vi "FFT.vi"() -> ()   [LabVIEW 2020]
uses:
  <vilib>/rvi/Analysis/measure/FFT/simModelSupport/niFPGA FFT Outside SCTL Sim Properties.ctl
  <vilib>/rvi/Analysis/measure/FFT/simModelSupport/niFPGA FFT Sim Types.ctl
  <vilib>/rvi/Analysis/measure/FFT/simModelSupport/niFpgaFFTSimArithmeticProperties.ctl
  <vilib>/rvi/Analysis/measure/FFT/simModelSupport/niFpgaFFTSimDfxp.ctl
  <vilib>/fxp/LVFixedPointQuantizationPolicyTypeDef.ctl
  <vilib>/rvi/FXPMathLib/FxpAtan2/subVIs/nifxpmath_Atan2_SimConfig.ctl
  <vilib>/rvi/FXPMathLib/FxpSinAndCos/subVIs/nifxpmath_SinAndCos_SimConfig.ctl
  <vilib>/rvi/DataTransferAndStorage/Container/Common/niFpgaContainerGetUniqueNameForEmu.vi
  <vilib>/rvi/DataTransferAndStorage/Container/Common/niFpgaContainerSetEmuInfo.vi
  <vilib>/rvi/eio/common/nirviEmuReportErrorAndStop.vi
  <vilib>/rvi/interface/RandomDataEmulation/niFpgaRandomDataHandleErrors.vi
  <vilib>/rvi/DataTransferAndStorage/Container/Common/niFpgaContainerExecOnDevCompGetState.vi
  <vilib>/rvi/Emulation/niFpgaEmulationIsFPGAContextNoSignature.vi
  <vilib>/rvi/Emulation/niFpgaSctlEmulationGetInTimedLoop.vi
  <vilib>/rvi/errors/niFpgaSetErrorForExecOnDevCompSimple.vi
  <vilib>/rvi/FIFO/Fifo_Resource/nirvififoEmulationSetSize.vi
  <vilib>/rvi/FIFO/Fifo_Resource/nirviFifoEmulationQueueMgr.vi
  <instcachedir>/0/nirviFifoEmulationQueueMgr_E5CAEC123FF24DC58D834DCA3CDAA9B5.lvgen/nirviFifoEmulationQueueMgr_E5CAEC123FF24DC58D834DCA3CDAA9B5_008.vi
  <vilib>/rvi/FIFO/Fifo_Resource/nirvififoEmulationDetermineInputValidOut.vi
  <vilib>/rvi/FIFO/Fifo_Resource/nirvififoEmulationCreateLock.vi
  <vilib>/rvi/Emulation/niFpgaProcessEmulError.vi
  <vilib>/rvi/FIFO/Fifo_Resource/nirvififoEmulationObtainLock.vi
  <vilib>/rvi/FIFO/Fifo_Resource/nirvififoEmulationReleaseLock.vi
  <vilib>/rvi/occurrence/nirviWaitOnOccurrenceBase.vi
  <vilib>/rvi/errors/nirviReportUnexpectedCaseInternalError.vi
  <vilib>/rvi/errors/nirviReportUnexpectedCaseInternalError (U32).vi
  <vilib>/Utility/error.llb/Clear Errors.vi
  <vilib>/rvi/Emulation/niFpgaGetClockAttributes.vi
  <vilib>/rvi/Emulation/niFpgaEmulationReportErrorSimple.vi
  <vilib>/rvi/Analysis/measure/FFT/simModelSupport/niFpgaFFTSimModelOutsideSCTLCore.vi
  <vilib>/rvi/FXPMathLib/FxpAtan2/simVIs/DllFxpAtan2Temp_sub.vi
  <instcachedir>/0/nirviFifoEmulationQueueMgr_E5CAEC123FF24DC58D834DCA3CDAA9B5.lvgen/nirviFifoEmulationQueueMgr_E5CAEC123FF24DC58D834DCA3CDAA9B5_002.vi
  <instcachedir>/0/nirviFifoEmulationQueueMgr_E5CAEC123FF24DC58D834DCA3CDAA9B5.lvgen/nirviFifoEmulationQueueMgr_E5CAEC123FF24DC58D834DCA3CDAA9B5_004.vi
  <vilib>/rvi/Emulation/niFpgaCriticalErrorInLSC.vi
  <vilib>/rvi/FXPMathLib/FxpSinAndCos/simVIs/DllFxpSinAndCosTemp_sub.vi
  <instcachedir>/0/nirviFifoEmulationQueueMgr_E5CAEC123FF24DC58D834DCA3CDAA9B5.lvgen/nirviFifoEmulationQueueMgr_E5CAEC123FF24DC58D834DCA3CDAA9B5_015.vi
  <vilib>/rvi/LocalResourceManager/LocalResourceManager.xnode
  <vilib>/rvi/DataTransferAndStorage/Container/XNode/niFpgaContainer.xnode
  <vilib>/rvi/interface/RandomDataEmulation/nirviRandomDataFpgaReadWriteTemplate.vi
  <vilib>/rvi/FIFO/Fifo_Resource/niFpgaFifoEmulationRefIn.vi
  <vilib>/rvi/Analysis/measure/FFT/XNode/niFpgaFFT.xnode
  <vilib>/rvi/FXPMathLib/FxpAtan2/XNode/nifxpmath_Atan2.xnode
  <vilib>/rvi/FXPMathLib/FxpSinAndCos/XNode/nifxpmath_SinAndCos.xnode
panel:
  out "Numeric 3":i32
  out "Numeric":i32
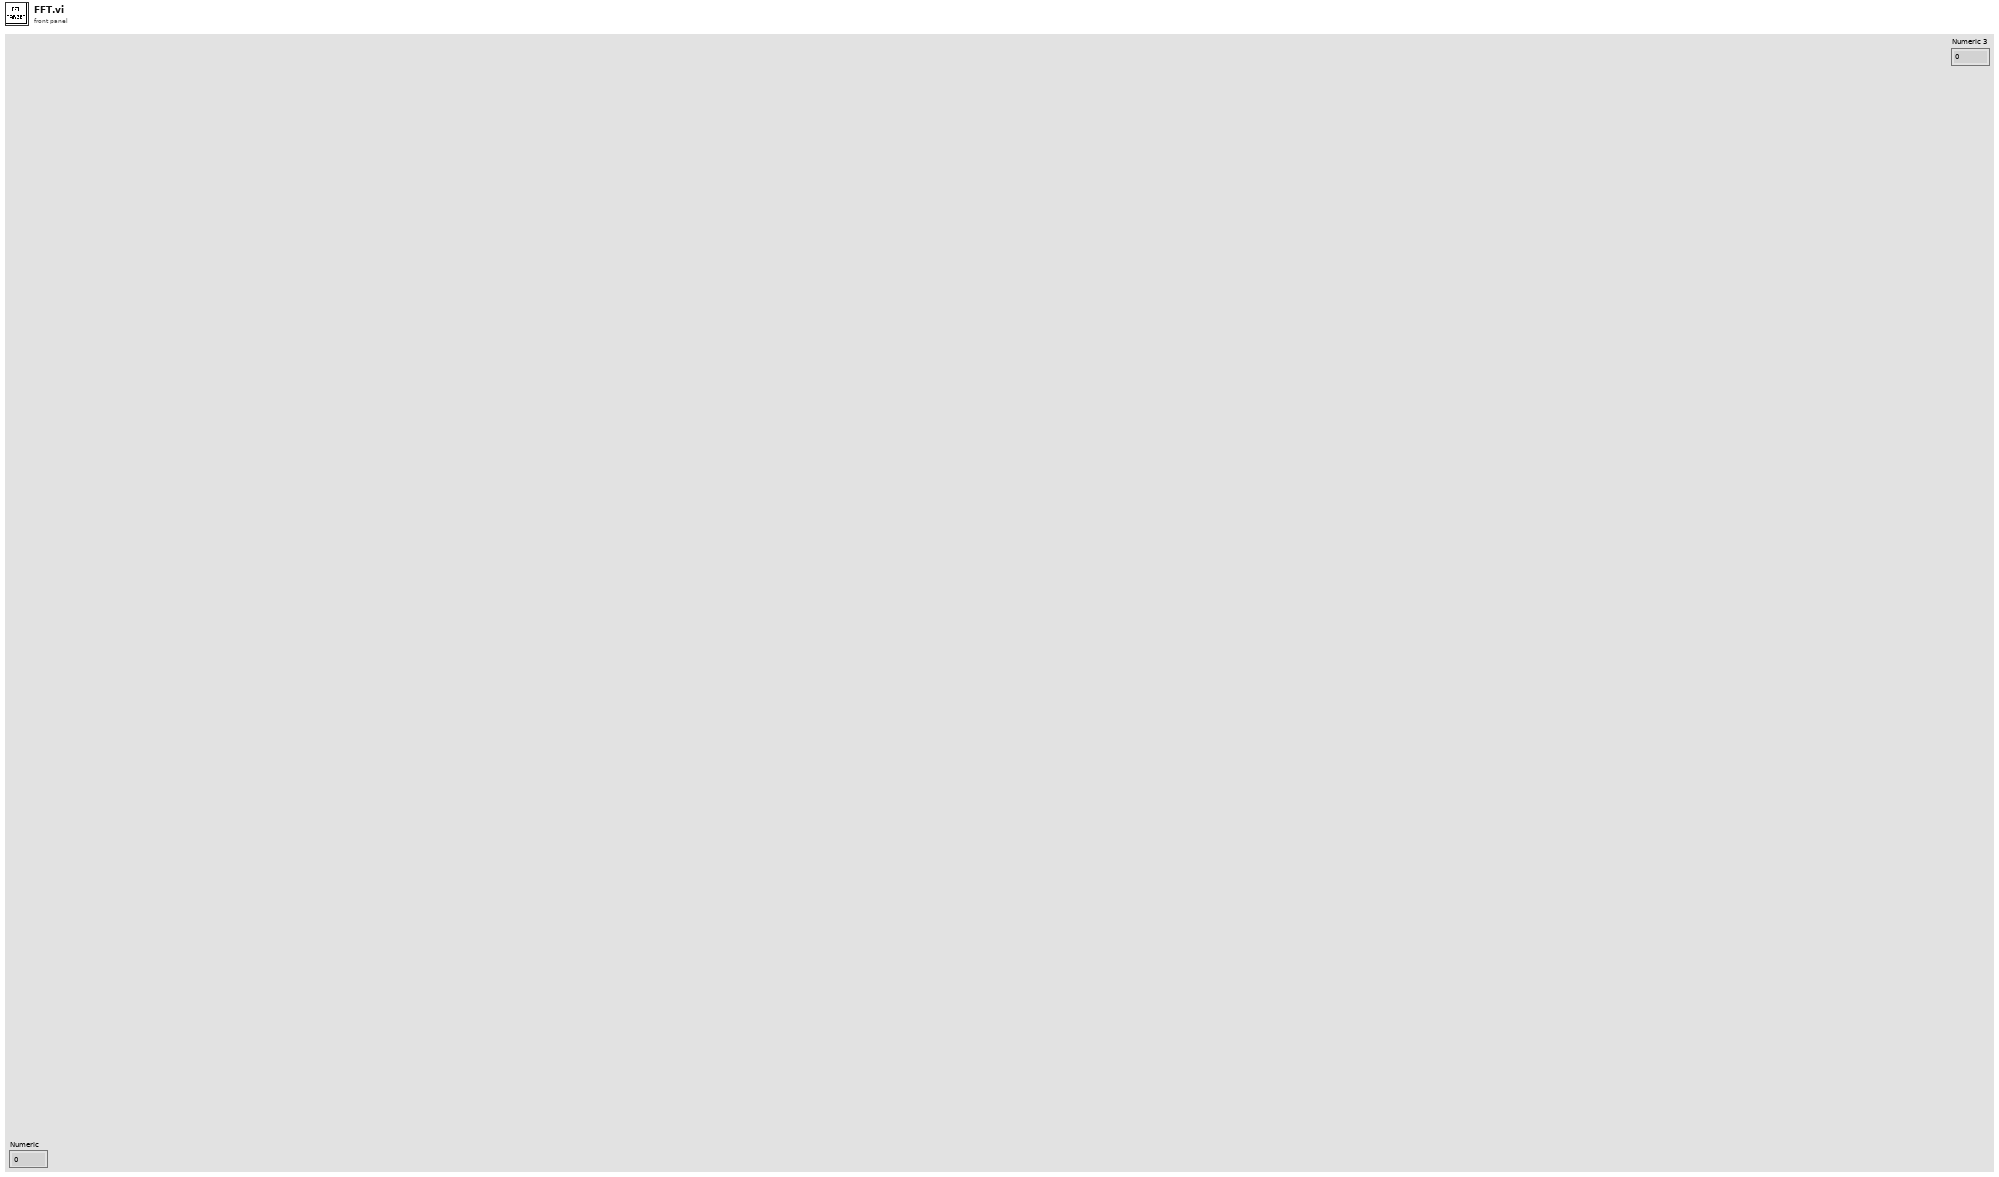
[diagram p1: front panel]
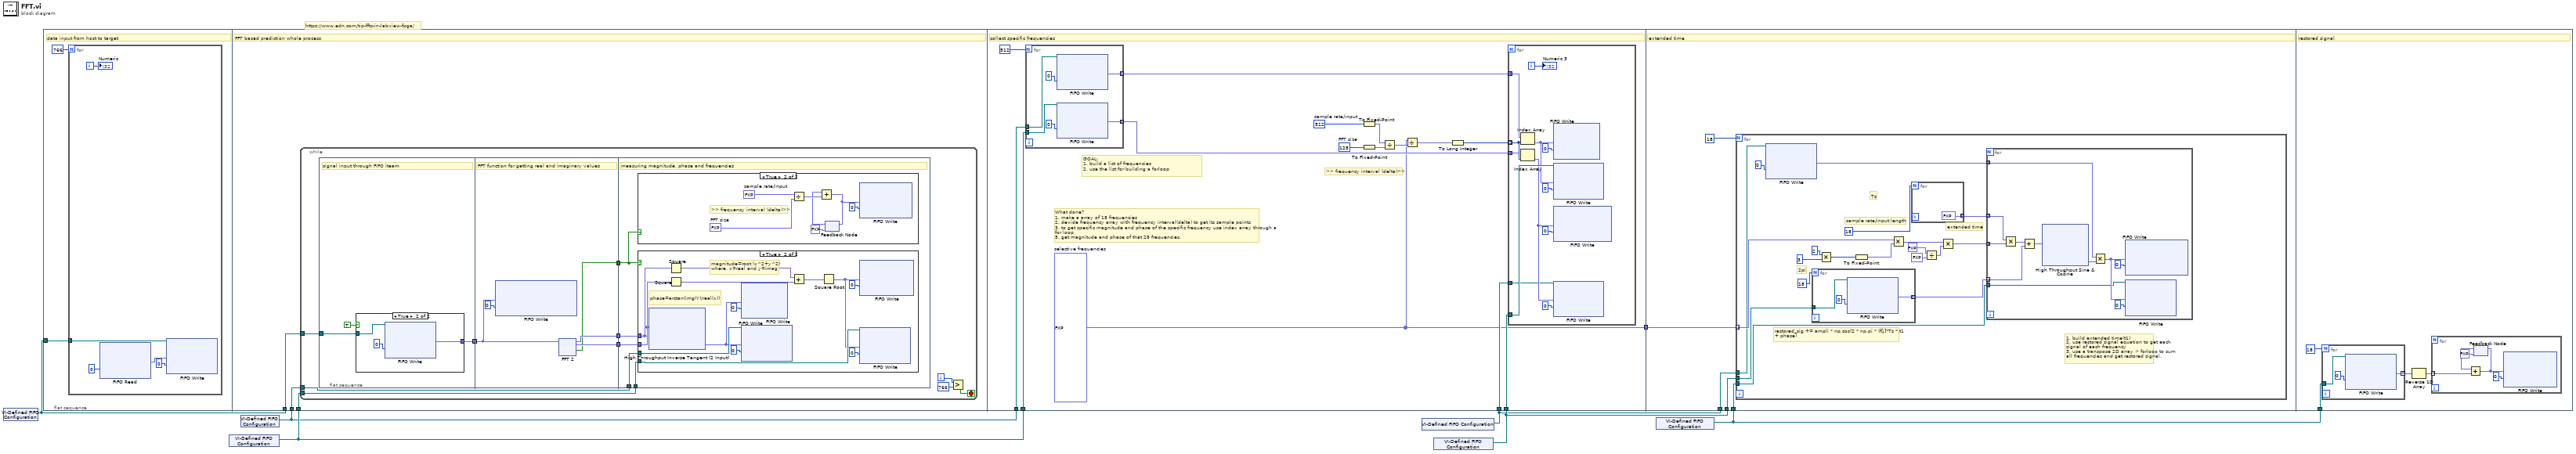
[diagram p0: block diagram]
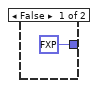
[diagram p2: hidden frame]
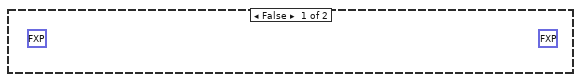
[diagram p4: hidden frame]
diagram:
  # "https://www.edn.com/tip-ffts-in-labview-fpga/"
  n1 = xnode "VI-Defined FIFO Configuration"() -> ("FIFO Out"=w7:refnum<k21>)
  n2 = flat-sequence {
    tunnel: w7 -> [w9]
    tunnel: w7 -> [w17]
    tunnel: w6 -> [w16]
    tunnel: w5 -> [w15]
    tunnel: w6 -> [w117]
    tunnel: w5 -> [w116]
    tunnel: w4 -> [w115]
    tunnel: w3 -> [w114]
    tunnel: [w113] -> w2
    tunnel: w4 -> [w150]
    tunnel: w3 -> [w149]
    tunnel: w2 -> [w148]
    tunnel: w1 -> [w147]
    tunnel: w1 -> [w218]
    frame #0 {
      # "data input from host to target"
      n3 = for {
        N: 766 -> [_]
        tunnel: w9 -> [w13]
        i -> [w10]
        n4 = xnode ("FIFO Read")("Timeout"=0) -> ("Element"=w11:fxp<+/-,24,7>)  [unwired: 1 in, 2 out]
        n5 = xnode ("FIFO Write")("Element"=w11, "Timeout"=0, "FIFO In"=w13) -> ()  [unwired: 2 out]
        "Numeric" <- w10
      }
    }
    frame #1 {
      # "FFT based prediction whole process"
      n6 = while {
        tunnel: w17 -> [w26]
        tunnel: w16 -> [w19]
        tunnel: w15 -> [w18]
        i -> [w25]
        stop <- w20 stop-if-true
        n7 = flat-sequence {
          tunnel: w26 -> [w30]
          tunnel: [w28] -> w24
          tunnel: w24 -> [w39]
          tunnel: [w38] -> w23
          tunnel: [w37] -> w22
          tunnel: [w36] -> w21
          tunnel: w23 -> [w63]
          tunnel: w22 -> [w62]
          tunnel: w21 -> [w64]
          tunnel: w19 -> [w61]
          tunnel: w18 -> [w60]
          frame #0 {
            # "signal input through FIFO iteam"
            n8 = case shown="True" TRUE {
              tunnel: w30 -> [_ w34]
              tunnel: [fxp<+/-,24,7> 0.0 ("Element") w32] -> w28
              frame False {
              }
              frame True {
                n9 = xnode ("FIFO Write")("Timeout"=0, "FIFO In"=w34) -> ("Element"=w32:fxp<+/-,24,7>)  [unwired: 2 out]
              }
            }
          }
          frame #1 {
            # "FFT function for getting real and imaginary values"
            n10 = xnode ("FIFO Write")("Element"=w39, "Timeout"=0) -> ()  [unwired: 1 in, 2 out]
            n11 = xnode ("FFT 2")("real data in"=w39) -> ("real data out"=w38:fxp<+/-,32,15>, "imaginary data out"=w37:fxp<+/-,32,15>, "output valid"=w36:bool)  [unwired: 2 in, 1 out]
          }
          frame #2 {
            # "measuring magnitude, phase and frequencies"
            n12 = case shown="True" w64 {
              frame False {
              }
              frame True {
                w66 = fxp<+,1,10> 512.0  # sample rate/input
                w65 = fxp<+,1,8> 128.0  # FFT size
                # ">> frequency interval (delta)>>"
                n13 = Divide(x=w66, y=w65) -> (x/y=w70:fxp<+/-,32,16>)
                n14 = feedback #1(fxp<+/-,32,16> 0.0) -> (w68:fxp<+/-,32,16>)
                n15 = Add(x=w68, y=w70) -> (x+y=w69:fxp<+/-,32,16>)
                n16 = feedback-in #1(w69) -> ()
                n17 = xnode ("FIFO Write")("Element"=w69, "Timeout"=0) -> ()  [unwired: 1 in, 2 out]
              }
            }
            n18 = case shown="True" w64 {
              tunnel: w62 -> [_ w74]
              tunnel: w63 -> [_ w73]
              tunnel: w61 -> [_ w78]
              tunnel: w60 -> [_ w75]
              frame False {
                (unwired) fxp<+/-,32,16> 0.0
                (unwired) fxp<+/-,32,16> 0.0
              }
              frame True {
                # "magnitude=root (x^2+y^2)\nwhere, x=real and y=imag"
                # "phase=arctan(img(Y)/real(x))"
                n19 = xnode "High Throughput Inverse Tangent (2 Input)"("y"=w74, "x"=w73) -> ("atan2(y,x) (pi)"=w72:fxp<+/-,16,2>)
                n20 = Square(x=w73) -> (x^2=w82:fxp<+,63,29>)
                n21 = Square(x=w74) -> (x^2=w77:fxp<+,63,29>)
                n22 = xnode ("FIFO Write")("Element"=w72, "Timeout"=0) -> ()  [unwired: 1 in, 2 out]
                n23 = xnode ("FIFO Write")("Element"=w72, "Timeout"=0, "FIFO In"=w75) -> ()  [unwired: 2 out]
                n24 = Add(x=w82, y=w77) -> (x+y=w81:fxp<+,64,30>)
                n25 = Square Root(x=w81) -> (sqrt(x)=w80:fxp<+/-,32,16>)
                n26 = xnode ("FIFO Write")("Element"=w80, "Timeout"=0) -> ()  [unwired: 1 in, 2 out]
                n27 = xnode ("FIFO Write")("Element"=w80, "Timeout"=0, "FIFO In"=w78) -> ()  [unwired: 2 out]
              }
            }
          }
        }
        n28 = Greater?(x=w25, y=766 ("Timeout")) -> (0:w20:bool)
      }
    }
    frame #2 {
      w122 = 512  # sample rate/input
      w123 = 128  # FFT size
      w113 = fxp<+/-,32,16>[] [128.0, 132.0, 136.0, 252.0, 256.0, 260.0, 380.0, 384.0, 388.0, -128.0, -132.0, -136.0, -252.0, -256.0, -260.0, -380.0, -384.0, -388.0]  # selective frequencies
      # "GOAL:\n1. build a list of frequencies\n2. use the list for building a forloop"
      # "What done?\n1. make a array of 18 frequencies\n2. devide frequency array with frequency interval(delta) to get its sample points\n3. to get specific magnitude and phase of the specific frequency use index array through a for loop\n5. get magnitude and phase of that 28 frequencies."
      # ">> frequency interval (delta)>>"
      # "collect specific frequencies"
      n29 = for {
        N: 512 -> [_]
        tunnel: [w143] -> w121 mode=indexing
        tunnel: [w142] -> w120 mode=indexing
        tunnel: w117 -> [w141]
        tunnel: w116 -> [w140]
        n30 = xnode ("FIFO Write")("Timeout"=0, "FIFO In"=w140) -> ("Element"=w143:fxp<+/-,16,2>)  [unwired: 2 out]
        n31 = xnode ("FIFO Write")("Timeout"=0, "FIFO In"=w141) -> ("Element"=w142:fxp<+/-,32,16>)  [unwired: 2 out]
      }
      n32 = To Fixed-Point(number=w122) -> (fixed-point=w125:fxp<+/-,32,32>)  [unwired: 1 in]
      n33 = To Fixed-Point(number=w123) -> (fixed-point=w124:fxp<+/-,32,32>)  [unwired: 1 in]
      n34 = Divide(x=w125, y=w124) -> (x/y=w126:fxp<+/-,32,16>)
      n35 = Divide(x=w113, y=w126) -> (x/y=w127:fxp<+/-,32,16>[])
      n36 = To Long Integer(number=w127) -> (32bit integer=w119:i32[])
      n37 = for {
        tunnel: w119 -> [w138] mode=indexing
        tunnel: w121 -> [w137]
        tunnel: w120 -> [w136]
        tunnel: w115 -> [w133]
        tunnel: w114 -> [w128]
        i -> [w139]
        n38 = Index Array(array=w137, index=w138) -> (element=w132:fxp<+/-,16,2>)
        n39 = Index Array(array=w136, index=w138) -> (element=w130:fxp<+/-,32,16>)
        n40 = xnode ("FIFO Write")("Element"=w132, "Timeout"=0) -> ()  [unwired: 1 in, 2 out]
        n41 = xnode ("FIFO Write")("Element"=w132, "Timeout"=0, "FIFO In"=w133) -> ()  [unwired: 2 out]
        n42 = xnode ("FIFO Write")("Element"=w130, "Timeout"=0) -> ()  [unwired: 1 in, 2 out]
        n43 = xnode ("FIFO Write")("Element"=w130, "Timeout"=0, "FIFO In"=w128) -> ()  [unwired: 2 out]
        "Numeric 3" <- w139
      }
    }
    frame #3 {
      # "extended time"
      n44 = for {
        N: 18 -> [_]
        tunnel: w150 -> [w169]
        tunnel: w149 -> [w157]
        tunnel: w148 -> [w168] mode=indexing
        tunnel: w147 -> [w161]
        # "extended time"
        # "sample rate/input length"
        # "Ts"
        # "1. build extended time(t1)\n2. use restored signal equation to get each signal of each frequency\n3. use a transpose 2D array > forloop to sum all frequencies and get restored signal."
        # "2pi"
        # "restored_sig += ampli * np.cos(2 * np.pi * (f[j]*Ts * t1 + phase)"
        n45 = xnode ("FIFO Write")("Timeout"=0, "FIFO In"=w157) -> ("Element"=w156:fxp<+/-,32,16>)  [unwired: 2 out]
        n46 = for {
          N: 18 -> [_]
          tunnel: w169 -> [w214]
          tunnel: [w212] -> w167 mode=indexing
          n47 = xnode ("FIFO Write")("Timeout"=0, "FIFO In"=w214) -> ("Element"=w212:fxp<+/-,16,2>)  [unwired: 2 out]
        }
        n48 = Multiply(x=2, y=3) -> (x*y=w164:i32)
        n49 = To Fixed-Point(number=w164) -> (fixed-point=w163:fxp<+/-,32,32>)  [unwired: 1 in]
        n50 = Multiply(x=w168, y=w163) -> (x*y=w154:fxp<+/-,64,48>)
        n51 = for {
          N: 18 -> [_]
          tunnel: [fxp<+,1,11> 1024.0 ("x")] -> w151 mode=indexing
        }
        n52 = Divide(x=fxp<+,1,1> 1.0 ("y"), y=fxp<+,1,10> 512.0) -> (x/y=w155:fxp<+/-,32,16>)
        n53 = Multiply(x=w154, y=w155) -> (x*y=w152:fxp<+/-,32,16>)
        n54 = for {
          tunnel: w167 -> [w181] mode=indexing
          tunnel: w156 -> [w174]
          tunnel: w161 -> [w176]
          tunnel: w152 -> [w173]
          tunnel: w151 -> [w171] mode=indexing
          n55 = Multiply(x=w171, y=w173) -> (x*y=w172:fxp<+/-,32,26>)
          n56 = Add(x=w172, y=w181) -> (x+y=w175:fxp<+/-,32,16>)
          n57 = xnode "High Throughput Sine & Cosine"("x (pi)"=w175) -> ("cos(x)"=w180:fxp<+/-,32,2>)  [unwired: 1 out]
          n58 = Multiply(x=w174, y=w180) -> (x*y=w178:fxp<+/-,64,18>)
          n59 = xnode ("FIFO Write")("Element"=w178, "Timeout"=0) -> ()  [unwired: 1 in, 2 out]
          n60 = xnode ("FIFO Write")("Element"=w178, "Timeout"=0, "FIFO In"=w176) -> ()  [unwired: 2 out]
        }
      }
    }
    frame #4 {
      # "restored signal"
      n61 = for {
        N: 18 -> [_]
        tunnel: w218 -> [w220]
        tunnel: [w219] -> w216 mode=indexing
        n62 = xnode ("FIFO Write")("Timeout"=0, "FIFO In"=w220) -> ("Element"=w219:fxp<+/-,64,18>)  [unwired: 2 out]
      }
      n63 = Reverse 1D Array(array=w216) -> (reversed array=w215:fxp<+/-,64,18>[])
      n64 = for {
        tunnel: w215 -> [w222] mode=indexing
        n65 = feedback #2(fxp<+/-,32,16> 0.0) -> (w226:fxp<+/-,32,16>)
        n66 = Add(x=w226, y=w222) -> (x+y=w224:fxp<+/-,32,16>)
        n67 = feedback-in #2(w224) -> ()
        n68 = xnode ("FIFO Write")("Element"=w224, "Timeout"=0) -> ()  [unwired: 1 in, 2 out]
      }
    }
  }
  n69 = xnode "VI-Defined FIFO Configuration"() -> ("FIFO Out"=w6:refnum<k21>)
  n70 = xnode "VI-Defined FIFO Configuration"() -> ("FIFO Out"=w5:refnum<k21>)
  n71 = xnode "VI-Defined FIFO Configuration"() -> ("FIFO Out"=w3:refnum<k21>)
  n72 = xnode "VI-Defined FIFO Configuration"() -> ("FIFO Out"=w4:refnum<k21>)
  n73 = xnode "VI-Defined FIFO Configuration"() -> ("FIFO Out"=w1:refnum<k21>)
